vi "GetTableRow.vi"(8 "error in (no error)":errorcluster, 11 "Table in":refnum<class "Table.lvclass">) -> (0 "error out":errorcluster, 2 "TableRow":refnum<class "Collection.lvclass">[](array[class]), 3 "Table out":refnum<class "Table.lvclass">)   [LabVIEW 2021, in "LvMarkdown.lvlib" / "Table.lvclass"]
uses:
  Table.lvclass
  Table.lvclass/Table.ctl
  Collection/Collection.lvclass
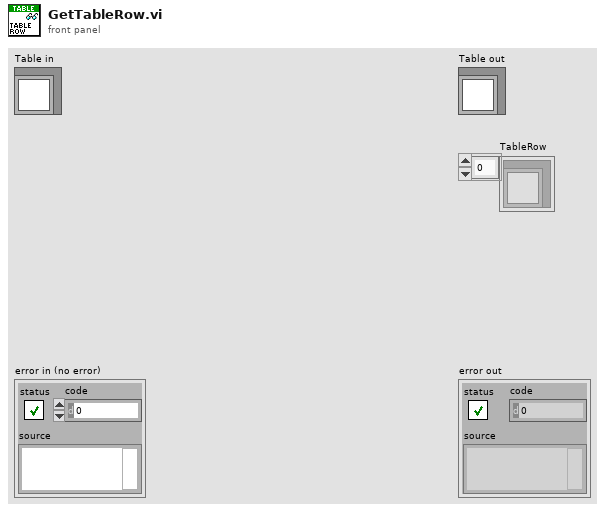
[diagram p1: front panel]
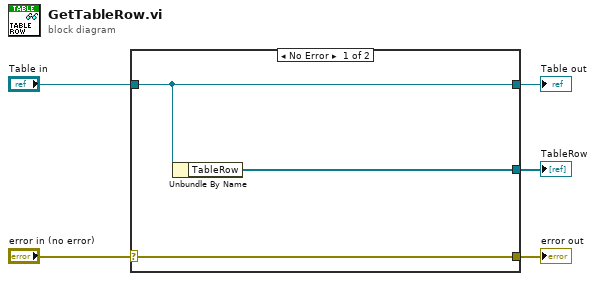
[diagram p0: block diagram]
diagram:
  n1 = case shown="No Error" "error in (no error)" {
    selector: "error in (no error)" -> [w8 w9]
    tunnel: [w8 w9] -> w4
    tunnel: [w7 w10] -> w2
    tunnel: "Table in" -> [w7 w10]
    tunnel: [w6 _] -> w1
    frame No Error {
      n2 = Unbundle By Name(w7) -> ("TableRow"=w6:refnum<class "Collection.lvclass">[])
    }
    frame Error {
    }
  }
  "error out" <- w4
  "Table out" <- w2
  "TableRow" <- w1
